vi "FTW-DevUtil-VIDetails.vi"() -> ()   [LabVIEW 2015]
uses:
  linker/FTW-Linker-LinkerInfoStructure.ctl
  linker/FTW-Linker-LabVIEWFiletype.ctl
  linker/FTW-Linker-Flags-viflags2.ctl
  linker/FTW-Linker-Flags-wStyle.ctl
  linker/FTW-Linker-Flags-buttons.ctl
  linker/FTW-Linker-Flags-iState.ctl
  linker/FTW-Linker-Flags-iStyle.ctl
  linker/FTW-Linker-Flags-viflags.ctl
  src/reflection/FTW-Reflection-Types.ctl
panel:
  in  "ScanCLFN":bool=TRUE
  out "CLFN Progress...":dbl(slide) scale=0.0..1.0
  out "Loading Progress...":dbl(slide) scale=0.0..1.0
  in  "Tab":T1(tab)
  in  "Target to Scan":T2(radio)
  out "All Contexts":string[](array[string])
  in  "Context Filter":string="My\\sComputer | XNode | .*"
  out "VIs":T3(array[cluster]) {"SaveVersion" format="%08x"; "FPFlags" format="%08x"; "BDFlags" format="%08x"; "Complexity" format="%.1f"; "HistoryRevision" format="rev %d"; "CompileTime" format="Compile: %dmsec"; "NumCallers" format="%d callers"; "CodeSize" format="BD: %06.1p"; "FPSize" format="FP: %06.1p"}
  in  "Order By":T4(ring)
  out "Controls":T5(array[cluster]) {"HistoryRevision" format="rev %d"; "Callers" format="%d callers"; "FPSize" format="FP %.1p"}
  in  "OrderByDocs":T6(ring) caption="Order By"
  out "VIDocs":T7(array[cluster])
  in  "ContextFilterDocs":string="My\\sComputer | XNode | .*"
  out "All Prototypes":string
  out "CLFNs":T8(array[cluster])
  out "All Links":cluster{"Name":string, "Path":string}[](array[cluster])
  out "LinkerInfo":T9[](array[typedef]) {"iState" format="%08x"; "iStyle" format="%08x"; "wStyle" format="%08x"; "buttons" format="%08x"; "viflags" format="%08x"; "viflags2" format="%08x"}
  out "ExtendedLinkerInfo":T11(array[cluster])
  out "Hover Tip":string
  out "Array":T12(array[cluster]) {"Percentage" format="%.3f%%"}
  in  "Check Coverage":bool
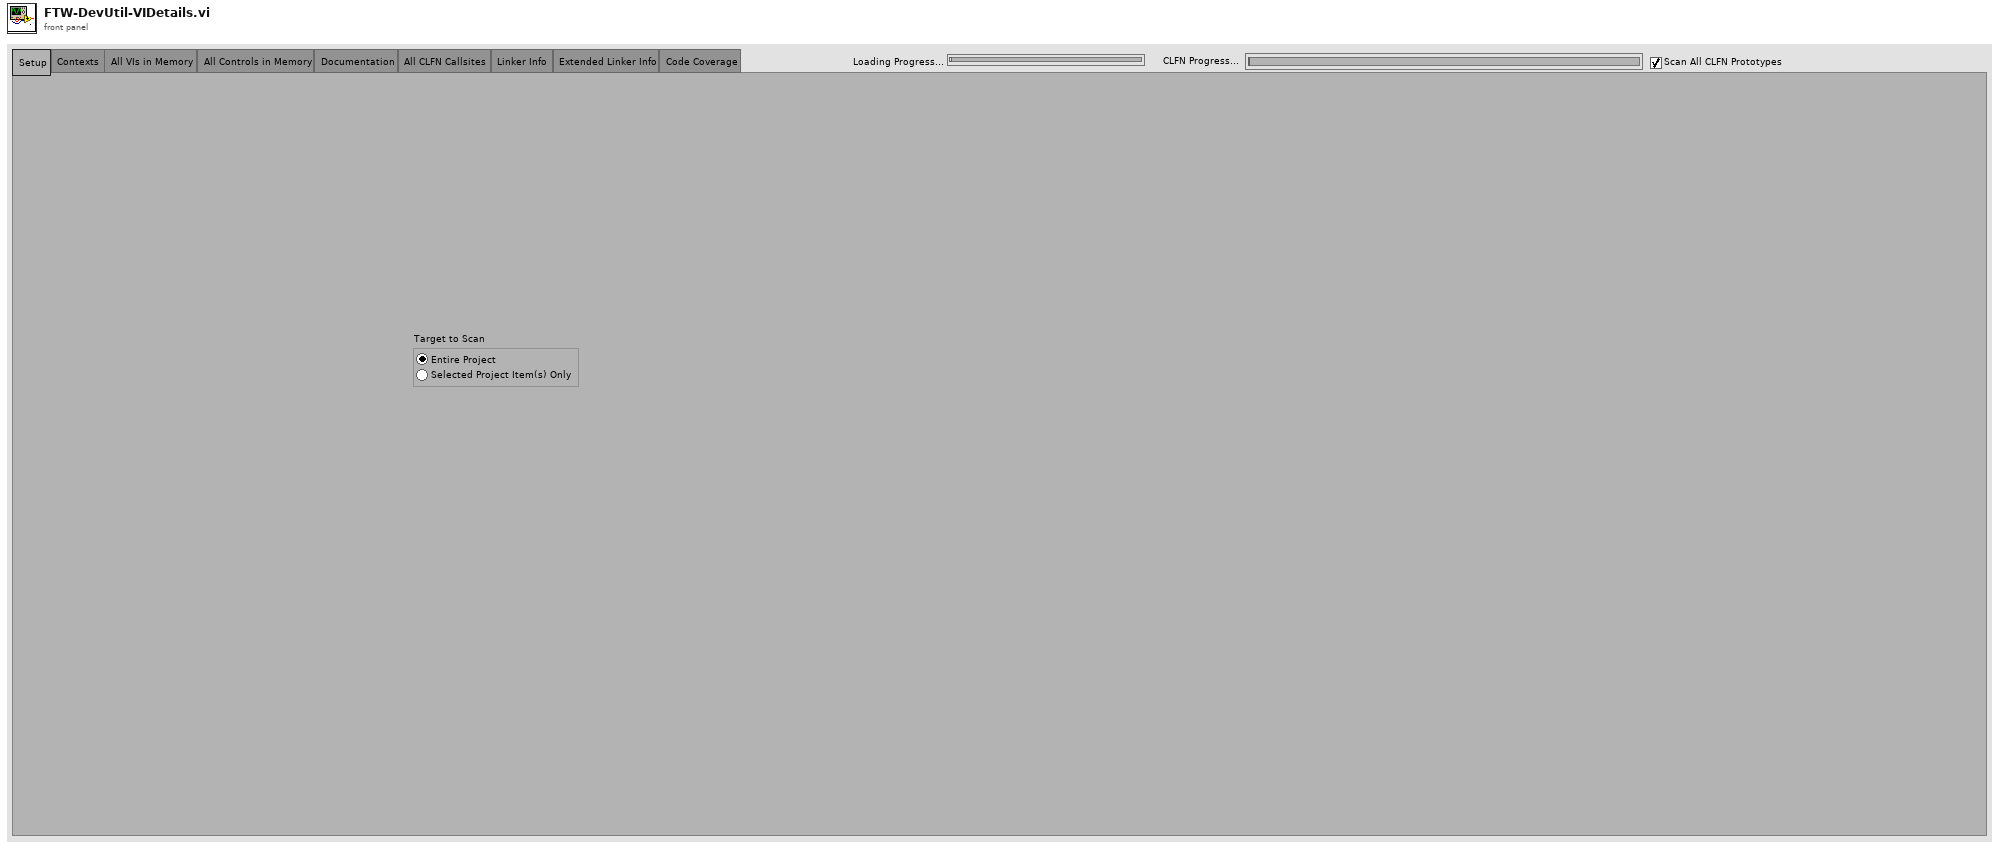
[diagram p1: front panel]
types:
  T1 = enum32{"Setup", "Contexts", "All VIs in Memory", "All Controls in Memory", "Documentation", "All CLFN Callsites", "Linker Info", "Extended Linker Info", "Code Coverage"}
  T2 = enum32{"Entire Project", "Selected Project Item Only"}
  T3 = cluster{"VIRef":refnum<vi>, "Context":string, "Name":string, "FPSize":u32, "CodeSize":u32, "NumCallers":i32, "CompileTime":i32, "Execution":string, "UnexpectedConfig":bool, "ShowRunButton":bool, "ShowRunContButton":bool, "HistoryRevision":u32, "Complexity":sgl, "BDFlags":u32, "FPFlags":u32, "SaveVersion":u32}[]
  T4 = enum16{"Application Context", "Num Callers", "Complexity", "Diagram Size", "FP Size", "Compile Time", "Revisions", "Execution Settings"}
  T5 = cluster{"VIRef":refnum<vi>, "Context":string, "VI":string, "FPSize":u32, "Callers":i32, "SeparateCompiled":bool, "HistoryRevision":u32}[]
  T6 = enum16{"Name", "ConPane Style", "Required Terminals", "Recommended Terminals", "Total Terminals"}
  T7 = cluster{"VIRef":refnum<vi>, "Icon":picture, "Name":string, "HasTags":bool, "VIDescription":string, "Icon16":picture, "IconMono":picture, "OnlineHelp":bool, "ConPane":u32, "Context":string, "InReq":u32, "OutReq":u32, "InRec":u32, "OutRec":u32, "InOpt":u32, "OutOpt":u32, "InDD":u32, "OutDD":u32, "Wired Terms":u32, "WindowTitle":string, "CustomTitle":bool}[]
  T8 = cluster{"CLFNRef":refnum<vi>, "VI":string, "Function":string, "Prototype":string, "CallConv":u32, "LibraryPath":path, "AnyThread":bool, "Dynamic":bool, "ErrCheckLevel":u32, "Reserve":string, "Unreserve":string, "Abort":string, "Prealloc":bool[], "Err":string}[]
  T9 = typedef "FTW-Linker-LinkerInfoStructure.ctl" = cluster{"path":path, "delimited name":string, "Filetype":T10, "iState":u32, "iStyle":u16, "wStyle":u16, "buttons":u16, "viflags":u32, "viflags2":u32, "links":u32[]}
  T10 = typedef "FTW-Linker-LabVIEWFiletype.ctl" = enum32{"Invalid file", "Unknown type", "VI", "Control", "PolyVI", "Project", "Library", "LVClass", "XControl", "XNode", "Shared Library", "dotNET assembly", "ActiveX interface", "CIN", "Run-time menu", "Palette menu", "Help file", "LLB", "XNode Edit Dependency", "LVClass Private Data", "Statechart", "MathScript .m file", "Ladder Diagram", "Packed Project Lib", "XNode Build Dependency"}
  T11 = cluster{"Name":string, "Type":string, "Flags":bool[], "VIRef":refnum<vi>}[]
  T12 = cluster{"Info":bool, "Percentage":dbl, "Path":string}[]
  T13 = typedef "FTW-Linker-Flags-viflags.ctl" = cluster{"Broken Wire":bool, "Broken Node":bool, "Missing SubVI Link":bool, "Broken SubVI":bool, "Not Reservable":bool, "Reentrant":bool, "Close afterward if originally closed":bool, "Reentrant (shared clones)":bool, "Load Front Panel when opened":bool, "Block Diagram not available":bool, "Show front panel when loaded":bool, "Must Call Parent contract broken":bool, "Suspend when called":bool, "Locked":bool, "Run when opened":bool, "Show Front Panel when Called":bool, "Could not compile":bool, "Subroutine priority":bool, "Auto-log at finish":bool, "Compiler bug":bool, "Is Typedef":bool, "Is Strict Typedef":bool, "Bad DDO":bool, "Control Editor has unapplied changes":bool, "Boolean 25":bool, "Owning library broken":bool, "Auto preallocate arrays and strings":bool, "Show Evaluation Watermark":bool, "Show Student Watermark":bool, "Insane VI":bool, "PropTypes warnings (maybe diagram disabled)":bool, "PolyVI broken":bool}
  T14 = typedef "FTW-Linker-Flags-iStyle.ctl" = cluster{"Horizonal Scrollbar Enabled":bool, "Vertical Scrollbar Enabled":bool, "Show menu bar":bool, "Show Toolbar when Running":bool, "Show menu bar":bool, "Window run-time position (Centered)":bool, "Window run-time position (Maximized)":bool, "Allow default run-time shortcut menus":bool, "Highlight Enter Button":bool, "Boolean 10":bool, "Maintain window proportions for different resolutions":bool, "Boolean 12":bool, "Boolean 13":bool, "Boolean 14":bool, "Boolean 15":bool, "Boolean 16":bool}
  T15 = typedef "FTW-Linker-Flags-iState.ctl" = cluster{"Retain Wire Values":bool, "Boolean 2":bool, "Boolean 3":bool, "Boolean 4":bool, "Contains CLFN (???)":bool, "Auto-log at finish":bool, "Boolean 7":bool, "Boolean 8":bool, "Boolean 9":bool, "Allow Debugging":bool, "Boolean 11":bool, "Boolean 12":bool, "Boolean 13":bool, "Boolean 14":bool, "Boolean 15":bool, "Print Logging Enabled":bool, "Boolean 17":bool, "Boolean 18":bool, "Boolean 19":bool, "Boolean 20":bool, "Boolean 21":bool, "Boolean 22":bool, "Boolean 23":bool, "Locked":bool, "Boolean 25":bool, "Boolean 26":bool, "Boolean 27":bool, "Boolean 28":bool, "Boolean 29":bool, "Has Breakpoint":bool, "Allow Debugging":bool, "Boolean 32":bool}
  T16 = typedef "FTW-Linker-Flags-buttons.ctl" = cluster{"Hide Run Button":bool, "Boolean 2":bool, "Boolean 3":bool, "Boolean 4":bool, "Boolean 5":bool, "Hide Run Continuously Button":bool, "Boolean 7":bool, "Hide Abort Button":bool, "Boolean 9":bool, "Boolean 10":bool, "Boolean 11":bool, "Boolean 12":bool, "Is Dynamic Dispatch":bool, "Amalgamation":bool, "Amalgamation Piece":bool, "Dynamic Dispatch Method":bool}
  T17 = typedef "FTW-Linker-Flags-wStyle.ctl" = cluster{"Modal Window":bool, "Floating Window":bool, "Window has title bar":bool, "Allow user to close window":bool, "Allow user to resize window":bool, "Allow user to minimize window":bool, "Window runs transparently":bool, "Boolean 8":bool, "Boolean 9":bool, "Floating Window":bool, "Hide floating window if LV is not active":bool, "Boolean 12":bool, "Boolean 13":bool, "Boolean 14":bool, "Boolean 15":bool, "Boolean 16":bool}
  T18 = typedef "FTW-Linker-Flags-viflags2.ctl" = cluster{"Tagged and not edited":bool, "Hide Instance VI on Drop":bool, "Is System VI":bool, "Is Visible VI (perhaps in hierwin)":bool, "Is XNode VI":bool, "Template Rename in progress":bool, "Transactions Disabled":bool, "Must Call Parent contract satisfied":bool, "Undo/Redo didn't change types":bool, "TypePropper says OK to inline":bool, "Separate Compiled Code":bool, "Inline SubVI if possible":bool, "Transaction is failing":bool, "Runtime SSE optimization enabled":bool, "Student-only VI":bool, "Evaluation-only VI":bool, "Enable PolyVI type adaptation":bool, "Inline":bool, "Need FPDSO recompile":bool, "Deprecated PolyVI":bool, "VI can pass LVClass to CLFN":bool, "Undo/Redo in progress":bool, "Show PolyVI instance icon":bool, "Show PolyVI instance selector":bool, "Clear indicators when called":bool, "Expand when dropped as a SubVI":bool, "No clone if Instance VI":bool, "Is Class Private Data Control":bool, "Is Instance VI":bool, "Enable automatic error handling":bool, "Remote Panel VI":bool, "Suppress Instance VI Halo":bool}
  T19 = cluster{"App.ContextName":string, "Name":string, "Reference":refnum<vi>}
  T20 = cluster{"App.ContextName":string, string, "vi reference":refnum<vi>}
  T21 = cluster{"App.ContextName":string, "Name":string, "Reference":refnum<vi>}[]
  T22 = cluster{"VIRef":refnum<vi>, "Context":string, "VI":string, "FPSize":u32, "Callers":i32, "SeparateCompiled":bool, "HistoryRevision":u32}
  T23 = cluster{"VIRef":refnum<vi>, "Context":string, "Name":string, "FPSize":u32, "CodeSize":u32, "NumCallers":i32, "CompileTime":i32, "Execution":string, "UnexpectedConfig":bool, "ShowRunButton":bool, "ShowRunContButton":bool, "HistoryRevision":u32, "Complexity":sgl, "BDFlags":u32, "FPFlags":u32, "SaveVersion":u32}
  T24 = cluster{"VIRef":refnum<vi>, "Icon":picture, "Name":string, "HasTags":bool, "VIDescription":string, "Icon16":picture, "IconMono":picture, "OnlineHelp":bool, "ConPane":u32, "Context":string, "InReq":u32, "OutReq":u32, "InRec":u32, "OutRec":u32, "InOpt":u32, "OutOpt":u32, "InDD":u32, "OutDD":u32, "Wired Terms":u32, "WindowTitle":string, "CustomTitle":bool}
  T25 = enum32{"invalid VI type", "Standard VI", "Control VI", "Global VI", "Polymorphic VI", "Configuration VI", "SubSystem", "Facade VI", "Method VI", "Statechart Diagram VI"}
  T26 = typedef "imagedata.ctl" = cluster{"image type":i32, "image depth":i32, "image":u8[], "mask":u8[], "colors":u32[], "Rectangle":cluster{"left":i16, "top":i16, "right":i16, "bottom":i16}}
  T27 = enum16{"Invalid Wire Rule", "Required", "Recommended", "Optional", "Dynamic Dispatch"}[]
  T28 = cluster{"[0]":u32, "[1]":u32, "[2]":u32, "[3]":u32, "[4]":u32, "[5]":u32, "[6]":u32, "[7]":u32}
  T29 = cluster{"HistoryRevision":u32, "FPSize":u32, "Callers":i32, "CodeSize":u32, "CompileTime":i32, "Reentrancy":string, "ExecSystem":enum32{"invalid execution system", "user interface", "standard", "instrument i/o", "data acquisition", "other 1", "other 2", "same as caller"}, "Priority":enum32{"invalid priority", "background priority", "normal priority", "above normal priority", "high priority", "time critical priority", "subroutine"}, "UnexpectedConfig":bool, "Debug":bool, "SeparateCompiled":bool, "AutoErrHand":bool, "Purgative":bool, "ShowRunButton":bool, "ShowRunContButton":bool, "Complexity":sgl, "BDFlags":u32, "FPFlags":u32}
  T30 = cluster{"Name":string, "Path":path, "Reference":refnum<vi>}
  T31 = cluster{"Name":string, "Path":path, "Reference":refnum<vi>}[]
  T32 = typedef "FTW-Reflection-Types.ctl" = enum16{"Unknown", "Void", "Array", "Cluster", "LVObject", "Boolean", "I8", "I16", "I32", "I64", "U8", "U16", "U32", "U64", "SGL", "DBL", "EXT", "CSG", "CDB", "CXT", "FXP", "EnumU8", "EnumU16", "EnumU32", "EnumU64", "SGLwithUnit", "DBLwithUnit", "EXTwithUnit", "CSGwithUnit", "CDBwithUnit", "CXTwithUnit", "String", "Path", "Picture", "Tag", "LVVariant", "Timestamp", "WaveformI8", "WaveformI16", "WaveformI32", "WaveformI64", "WaveformU8", "WaveformU16", "WaveformU32", "WaveformU64", "WaveformSGL", "WaveformDBL", "WaveformEXT", "WaveformCSG", "WaveformCDB", "WaveformCXT", "WaveformDigital", "WaveformUnknownType", "DigitalData", "DynamicData", "ExternalData", "FileByteStream", "TDMStream", "dotNET", "ActiveX", "VIServerReference", "VIReference", "ApplicationInstance", "Menu", "ConnectionDataSocket", "ConnectionVISA", "ConnectionBluetooth", "ConnectionIrDA", "ConnectionTCP", "ConnectionUDP", "ConnectionHTTPClient", "ConnectionFTP", "Occurrence", "Notifier", "Queue", "Rendezvous", "Semaphore", "RTFIFO", "EventPublisher", "EventRegistration", "EventCallback", "DataValueReference", "GenericClass", "GenericClassTag", "GenericClassDeepCopy", "GenericClassFlattened", "GenericClassTagFlattened", "GenericReferenceType", "WindowsRegistry", "OverloadedDatalogRef", "ReferenceUnknownType", "ByteArray", "ConPaneInterface", "FTWObject"}
  T33 = cluster{"Element Name":string, "Element Type":T32, "Element Value":variant}[]
  T34 = cluster{"CLFNRef":refnum<vi>, "VI":string, "Function":string, "Prototype":string, "CallConv":u32, "LibraryPath":path, "AnyThread":bool, "Dynamic":bool, "ErrCheckLevel":u32, "Reserve":string, "Unreserve":string, "Abort":string, "Prealloc":bool[], "Err":string}
  T35 = cluster{"Context":string, "Name":string, "VIDetails":cluster{"VIRef":refnum<vi>, "Context":string, "Name":string, "FPSize":u32, "CodeSize":u32, "NumCallers":i32, "CompileTime":i32, "Execution":string, "UnexpectedConfig":bool, "ShowRunButton":bool, "ShowRunContButton":bool, "HistoryRevision":u32, "Complexity":sgl, "BDFlags":u32, "FPFlags":u32, "SaveVersion":u32}}
  T36 = cluster{"Context":string, "Name":string, "VIDetails":cluster{"VIRef":refnum<vi>, "Context":string, "Name":string, "FPSize":u32, "CodeSize":u32, "NumCallers":i32, "CompileTime":i32, "Execution":string, "UnexpectedConfig":bool, "ShowRunButton":bool, "ShowRunContButton":bool, "HistoryRevision":u32, "Complexity":sgl, "BDFlags":u32, "FPFlags":u32, "SaveVersion":u32}}[]
  T37 = cluster{"NumCallers":i32, "Name":string, "VIDetails":cluster{"VIRef":refnum<vi>, "Context":string, "Name":string, "FPSize":u32, "CodeSize":u32, "NumCallers":i32, "CompileTime":i32, "Execution":string, "UnexpectedConfig":bool, "ShowRunButton":bool, "ShowRunContButton":bool, "HistoryRevision":u32, "Complexity":sgl, "BDFlags":u32, "FPFlags":u32, "SaveVersion":u32}}
  T38 = cluster{"NumCallers":i32, "Name":string, "VIDetails":cluster{"VIRef":refnum<vi>, "Context":string, "Name":string, "FPSize":u32, "CodeSize":u32, "NumCallers":i32, "CompileTime":i32, "Execution":string, "UnexpectedConfig":bool, "ShowRunButton":bool, "ShowRunContButton":bool, "HistoryRevision":u32, "Complexity":sgl, "BDFlags":u32, "FPFlags":u32, "SaveVersion":u32}}[]
  T39 = cluster{"Complexity":sgl, "CodeSize":u32, "VIDetails":cluster{"VIRef":refnum<vi>, "Context":string, "Name":string, "FPSize":u32, "CodeSize":u32, "NumCallers":i32, "CompileTime":i32, "Execution":string, "UnexpectedConfig":bool, "ShowRunButton":bool, "ShowRunContButton":bool, "HistoryRevision":u32, "Complexity":sgl, "BDFlags":u32, "FPFlags":u32, "SaveVersion":u32}}
  T40 = cluster{"Complexity":sgl, "CodeSize":u32, "VIDetails":cluster{"VIRef":refnum<vi>, "Context":string, "Name":string, "FPSize":u32, "CodeSize":u32, "NumCallers":i32, "CompileTime":i32, "Execution":string, "UnexpectedConfig":bool, "ShowRunButton":bool, "ShowRunContButton":bool, "HistoryRevision":u32, "Complexity":sgl, "BDFlags":u32, "FPFlags":u32, "SaveVersion":u32}}[]
  T41 = cluster{"CodeSize":u32, "FPSize":u32, "VIDetails":cluster{"VIRef":refnum<vi>, "Context":string, "Name":string, "FPSize":u32, "CodeSize":u32, "NumCallers":i32, "CompileTime":i32, "Execution":string, "UnexpectedConfig":bool, "ShowRunButton":bool, "ShowRunContButton":bool, "HistoryRevision":u32, "Complexity":sgl, "BDFlags":u32, "FPFlags":u32, "SaveVersion":u32}}
  T42 = cluster{"CodeSize":u32, "FPSize":u32, "VIDetails":cluster{"VIRef":refnum<vi>, "Context":string, "Name":string, "FPSize":u32, "CodeSize":u32, "NumCallers":i32, "CompileTime":i32, "Execution":string, "UnexpectedConfig":bool, "ShowRunButton":bool, "ShowRunContButton":bool, "HistoryRevision":u32, "Complexity":sgl, "BDFlags":u32, "FPFlags":u32, "SaveVersion":u32}}[]
  T43 = cluster{"FPSize":u32, "CodeSize":u32, "VIDetails":cluster{"VIRef":refnum<vi>, "Context":string, "Name":string, "FPSize":u32, "CodeSize":u32, "NumCallers":i32, "CompileTime":i32, "Execution":string, "UnexpectedConfig":bool, "ShowRunButton":bool, "ShowRunContButton":bool, "HistoryRevision":u32, "Complexity":sgl, "BDFlags":u32, "FPFlags":u32, "SaveVersion":u32}}
  T44 = cluster{"FPSize":u32, "CodeSize":u32, "VIDetails":cluster{"VIRef":refnum<vi>, "Context":string, "Name":string, "FPSize":u32, "CodeSize":u32, "NumCallers":i32, "CompileTime":i32, "Execution":string, "UnexpectedConfig":bool, "ShowRunButton":bool, "ShowRunContButton":bool, "HistoryRevision":u32, "Complexity":sgl, "BDFlags":u32, "FPFlags":u32, "SaveVersion":u32}}[]
  T45 = cluster{"CompileTime":i32, "Name":string, "VIDetails":cluster{"VIRef":refnum<vi>, "Context":string, "Name":string, "FPSize":u32, "CodeSize":u32, "NumCallers":i32, "CompileTime":i32, "Execution":string, "UnexpectedConfig":bool, "ShowRunButton":bool, "ShowRunContButton":bool, "HistoryRevision":u32, "Complexity":sgl, "BDFlags":u32, "FPFlags":u32, "SaveVersion":u32}}
  T46 = cluster{"CompileTime":i32, "Name":string, "VIDetails":cluster{"VIRef":refnum<vi>, "Context":string, "Name":string, "FPSize":u32, "CodeSize":u32, "NumCallers":i32, "CompileTime":i32, "Execution":string, "UnexpectedConfig":bool, "ShowRunButton":bool, "ShowRunContButton":bool, "HistoryRevision":u32, "Complexity":sgl, "BDFlags":u32, "FPFlags":u32, "SaveVersion":u32}}[]
  T47 = cluster{"HistoryRevision":u32, "Name":string, "VIDetails":cluster{"VIRef":refnum<vi>, "Context":string, "Name":string, "FPSize":u32, "CodeSize":u32, "NumCallers":i32, "CompileTime":i32, "Execution":string, "UnexpectedConfig":bool, "ShowRunButton":bool, "ShowRunContButton":bool, "HistoryRevision":u32, "Complexity":sgl, "BDFlags":u32, "FPFlags":u32, "SaveVersion":u32}}
  T48 = cluster{"HistoryRevision":u32, "Name":string, "VIDetails":cluster{"VIRef":refnum<vi>, "Context":string, "Name":string, "FPSize":u32, "CodeSize":u32, "NumCallers":i32, "CompileTime":i32, "Execution":string, "UnexpectedConfig":bool, "ShowRunButton":bool, "ShowRunContButton":bool, "HistoryRevision":u32, "Complexity":sgl, "BDFlags":u32, "FPFlags":u32, "SaveVersion":u32}}[]
  T49 = cluster{"Execution":string, "Name":string, "VIDetails":cluster{"VIRef":refnum<vi>, "Context":string, "Name":string, "FPSize":u32, "CodeSize":u32, "NumCallers":i32, "CompileTime":i32, "Execution":string, "UnexpectedConfig":bool, "ShowRunButton":bool, "ShowRunContButton":bool, "HistoryRevision":u32, "Complexity":sgl, "BDFlags":u32, "FPFlags":u32, "SaveVersion":u32}}
  T50 = cluster{"Execution":string, "Name":string, "VIDetails":cluster{"VIRef":refnum<vi>, "Context":string, "Name":string, "FPSize":u32, "CodeSize":u32, "NumCallers":i32, "CompileTime":i32, "Execution":string, "UnexpectedConfig":bool, "ShowRunButton":bool, "ShowRunContButton":bool, "HistoryRevision":u32, "Complexity":sgl, "BDFlags":u32, "FPFlags":u32, "SaveVersion":u32}}[]
  T51 = cluster{"Context":string, "Name":string, "VIDocs":cluster{"VIRef":refnum<vi>, "Icon":picture, "Name":string, "HasTags":bool, "VIDescription":string, "Icon16":picture, "IconMono":picture, "OnlineHelp":bool, "ConPane":u32, "Context":string, "InReq":u32, "OutReq":u32, "InRec":u32, "OutRec":u32, "InOpt":u32, "OutOpt":u32, "InDD":u32, "OutDD":u32, "Wired Terms":u32, "WindowTitle":string, "CustomTitle":bool}}
  T52 = cluster{"Context":string, "Name":string, "VIDocs":cluster{"VIRef":refnum<vi>, "Icon":picture, "Name":string, "HasTags":bool, "VIDescription":string, "Icon16":picture, "IconMono":picture, "OnlineHelp":bool, "ConPane":u32, "Context":string, "InReq":u32, "OutReq":u32, "InRec":u32, "OutRec":u32, "InOpt":u32, "OutOpt":u32, "InDD":u32, "OutDD":u32, "Wired Terms":u32, "WindowTitle":string, "CustomTitle":bool}}[]
  T53 = cluster{"ConPane":u32, "Context":string, "Name":string, "VIDocs":cluster{"VIRef":refnum<vi>, "Icon":picture, "Name":string, "HasTags":bool, "VIDescription":string, "Icon16":picture, "IconMono":picture, "OnlineHelp":bool, "ConPane":u32, "Context":string, "InReq":u32, "OutReq":u32, "InRec":u32, "OutRec":u32, "InOpt":u32, "OutOpt":u32, "InDD":u32, "OutDD":u32, "Wired Terms":u32, "WindowTitle":string, "CustomTitle":bool}}
  T54 = cluster{"ConPane":u32, "Context":string, "Name":string, "VIDocs":cluster{"VIRef":refnum<vi>, "Icon":picture, "Name":string, "HasTags":bool, "VIDescription":string, "Icon16":picture, "IconMono":picture, "OnlineHelp":bool, "ConPane":u32, "Context":string, "InReq":u32, "OutReq":u32, "InRec":u32, "OutRec":u32, "InOpt":u32, "OutOpt":u32, "InDD":u32, "OutDD":u32, "Wired Terms":u32, "WindowTitle":string, "CustomTitle":bool}}[]
  T55 = cluster{u32, u32, "Name":string, "VIDocs":cluster{"VIRef":refnum<vi>, "Icon":picture, "Name":string, "HasTags":bool, "VIDescription":string, "Icon16":picture, "IconMono":picture, "OnlineHelp":bool, "ConPane":u32, "Context":string, "InReq":u32, "OutReq":u32, "InRec":u32, "OutRec":u32, "InOpt":u32, "OutOpt":u32, "InDD":u32, "OutDD":u32, "Wired Terms":u32, "WindowTitle":string, "CustomTitle":bool}}
  T56 = cluster{u32, u32, "Name":string, "VIDocs":cluster{"VIRef":refnum<vi>, "Icon":picture, "Name":string, "HasTags":bool, "VIDescription":string, "Icon16":picture, "IconMono":picture, "OnlineHelp":bool, "ConPane":u32, "Context":string, "InReq":u32, "OutReq":u32, "InRec":u32, "OutRec":u32, "InOpt":u32, "OutOpt":u32, "InDD":u32, "OutDD":u32, "Wired Terms":u32, "WindowTitle":string, "CustomTitle":bool}}[]
  T57 = cluster{"Wired Terms":u32, "Name":string, "VIDocs":cluster{"VIRef":refnum<vi>, "Icon":picture, "Name":string, "HasTags":bool, "VIDescription":string, "Icon16":picture, "IconMono":picture, "OnlineHelp":bool, "ConPane":u32, "Context":string, "InReq":u32, "OutReq":u32, "InRec":u32, "OutRec":u32, "InOpt":u32, "OutOpt":u32, "InDD":u32, "OutDD":u32, "Wired Terms":u32, "WindowTitle":string, "CustomTitle":bool}}
  T58 = cluster{"Wired Terms":u32, "Name":string, "VIDocs":cluster{"VIRef":refnum<vi>, "Icon":picture, "Name":string, "HasTags":bool, "VIDescription":string, "Icon16":picture, "IconMono":picture, "OnlineHelp":bool, "ConPane":u32, "Context":string, "InReq":u32, "OutReq":u32, "InRec":u32, "OutRec":u32, "InOpt":u32, "OutOpt":u32, "InDD":u32, "OutDD":u32, "Wired Terms":u32, "WindowTitle":string, "CustomTitle":bool}}[]
  T59 = cluster{"infoFound":bool, "covPercent":dbl, string}
  T60 = cluster{"infoFound":bool, "covPercent":dbl, string}[]
  T61 = cluster{string, "delimited name":string, "All Flags":bool[], "vi reference":refnum<vi>}
  T62 = cluster{"LibraryPath":path, "VI":string, "Function":string, "CLFN Array Element":cluster{"CLFNRef":refnum<vi>, "VI":string, "Function":string, "Prototype":string, "CallConv":u32, "LibraryPath":path, "AnyThread":bool, "Dynamic":bool, "ErrCheckLevel":u32, "Reserve":string, "Unreserve":string, "Abort":string, "Prealloc":bool[], "Err":string}}
  T63 = cluster{string, "delimited name":string, "All Flags":bool[], "vi reference":refnum<vi>}[]
  T64 = cluster{"LibraryPath":path, "VI":string, "Function":string, "CLFN Array Element":cluster{"CLFNRef":refnum<vi>, "VI":string, "Function":string, "Prototype":string, "CallConv":u32, "LibraryPath":path, "AnyThread":bool, "Dynamic":bool, "ErrCheckLevel":u32, "Reserve":string, "Unreserve":string, "Abort":string, "Prealloc":bool[], "Err":string}}[]
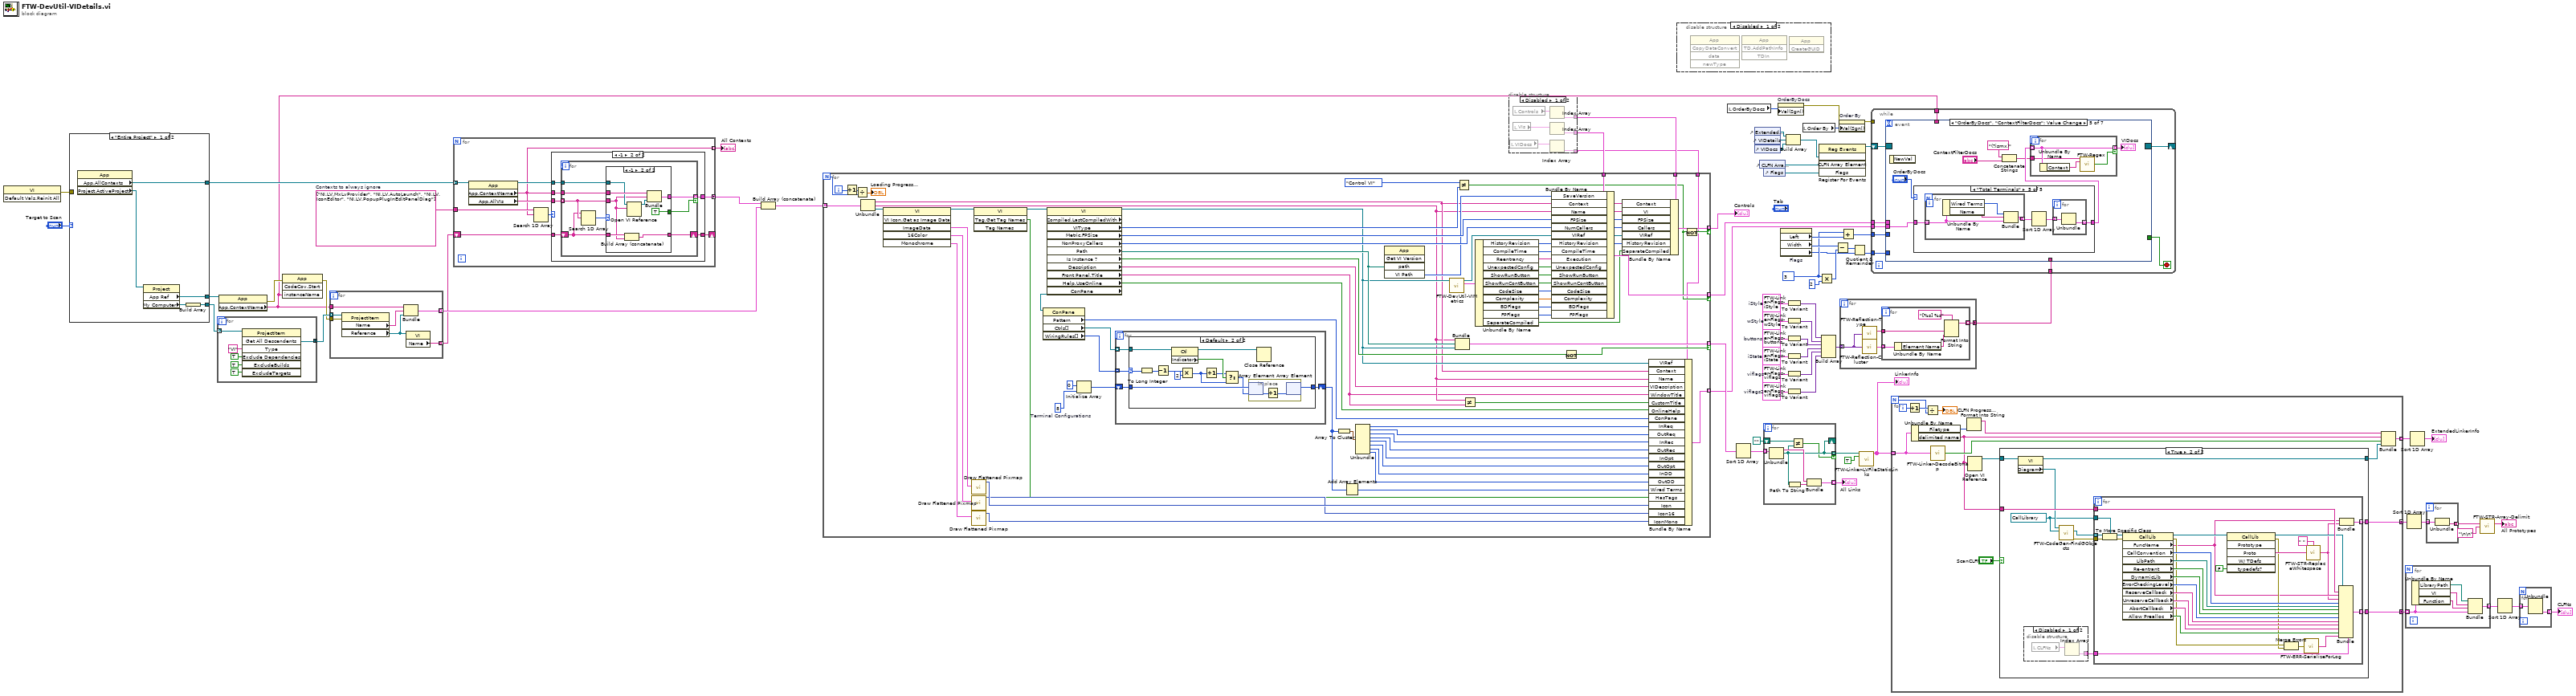
[diagram p0: block diagram]
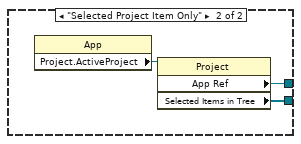
[diagram p3: hidden frame]
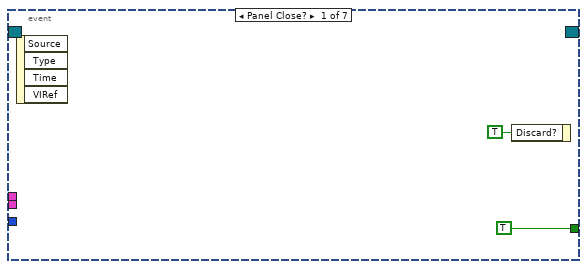
[diagram p8: hidden frame]
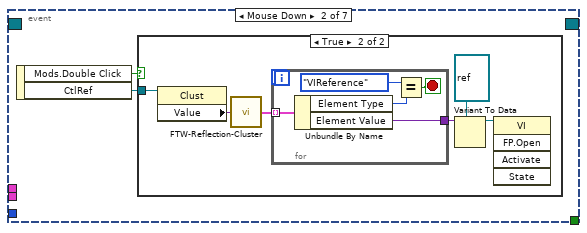
[diagram p9: hidden frame]
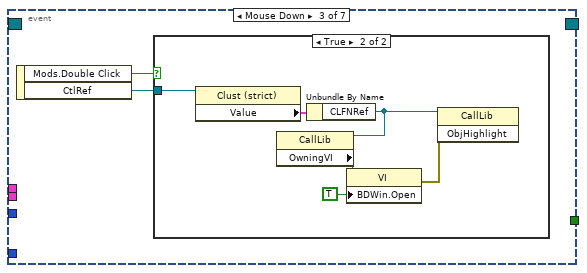
[diagram p11: hidden frame]
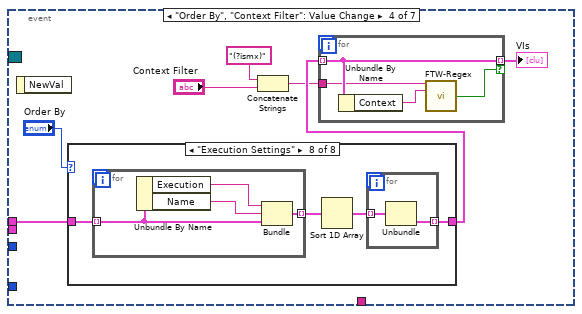
[diagram p13: hidden frame]
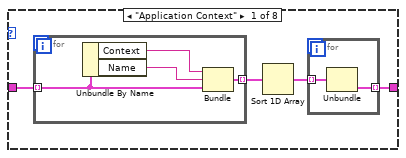
[diagram p14: hidden frame]
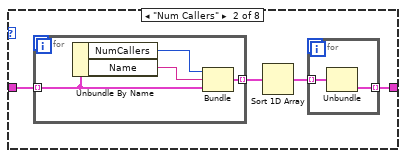
[diagram p15: hidden frame]
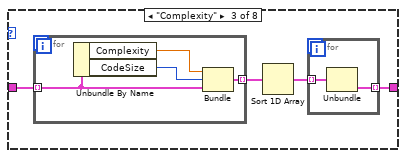
[diagram p16: hidden frame]
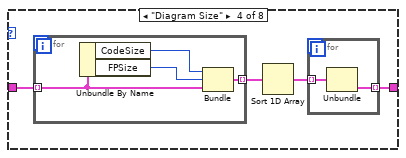
[diagram p17: hidden frame]
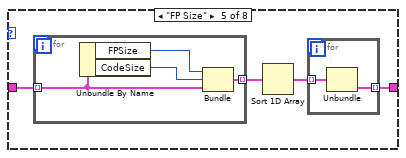
[diagram p18: hidden frame]
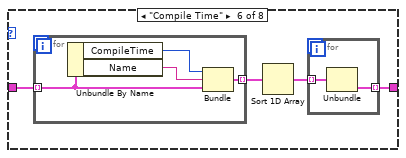
[diagram p19: hidden frame]
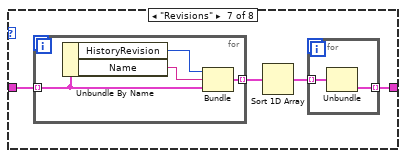
[diagram p20: hidden frame]
diagram:
  w21 = T13 {"Broken Wire"=FALSE, "Broken Node"=FALSE, "Missing SubVI Link"=FALSE, "Broken SubVI"=FALSE, "Not Reservable"=FALSE, "Reentrant"=FALSE, "Close afterward if originally closed"=FALSE, "Reentrant (shared clones)"=FALSE, "Load Front Panel when opened"=FALSE, "Block Diagram not available"=FALSE, "Show front panel when loaded"=FALSE, "Must Call Parent contract broken"=FALSE, "Suspend when called"=FALSE, "Locked"=FALSE, "Run when opened"=FALSE, "Show Front Panel when Called"=FALSE, "Could not compile"=FALSE, "Subroutine priority"=FALSE, "Auto-log at finish"=FALSE, "Compiler bug"=FALSE, "Is Typedef"=FALSE, "Is Strict Typedef"=FALSE, "Bad DDO"=FALSE, "Control Editor has unapplied changes"=FALSE, "Boolean 25"=FALSE, "Owning library broken"=FALSE, "Auto preallocate arrays and strings"=FALSE, "Show Evaluation Watermark"=FALSE, "Show Student Watermark"=FALSE, "Insane VI"=FALSE, "PropTypes warnings (maybe diagram disabled)"=FALSE, "PolyVI broken"=FALSE}  # viflags
  w25 = T14 {"Horizonal Scrollbar Enabled"=FALSE, "Vertical Scrollbar Enabled"=FALSE, "Show menu bar"=FALSE, "Show Toolbar when Running"=FALSE, "Show menu bar"=FALSE, "Window run-time position (Centered)"=FALSE, "Window run-time position (Maximized)"=FALSE, "Allow default run-time shortcut menus"=FALSE, "Highlight Enter Button"=FALSE, "Boolean 10"=FALSE, "Maintain window proportions for different resolutions"=FALSE, "Boolean 12"=FALSE, "Boolean 13"=FALSE, "Boolean 14"=FALSE, "Boolean 15"=FALSE, "Boolean 16"=FALSE}  # iStyle
  w22 = T15 {"Retain Wire Values"=FALSE, "Boolean 2"=FALSE, "Boolean 3"=FALSE, "Boolean 4"=FALSE, "Contains CLFN (???)"=FALSE, "Auto-log at finish"=FALSE, "Boolean 7"=FALSE, "Boolean 8"=FALSE, "Boolean 9"=FALSE, "Allow Debugging"=FALSE, "Boolean 11"=FALSE, "Boolean 12"=FALSE, "Boolean 13"=FALSE, "Boolean 14"=FALSE, "Boolean 15"=FALSE, "Print Logging Enabled"=FALSE, "Boolean 17"=FALSE, "Boolean 18"=FALSE, "Boolean 19"=FALSE, "Boolean 20"=FALSE, "Boolean 21"=FALSE, "Boolean 22"=FALSE, "Boolean 23"=FALSE, "Locked"=FALSE, "Boolean 25"=FALSE, "Boolean 26"=FALSE, "Boolean 27"=FALSE, "Boolean 28"=FALSE, "Boolean 29"=FALSE, "Has Breakpoint"=FALSE, "Allow Debugging"=FALSE, "Boolean 32"=FALSE}  # iState
  w23 = T16 {"Hide Run Button"=FALSE, "Boolean 2"=FALSE, "Boolean 3"=FALSE, "Boolean 4"=FALSE, "Boolean 5"=FALSE, "Hide Run Continuously Button"=FALSE, "Boolean 7"=FALSE, "Hide Abort Button"=FALSE, "Boolean 9"=FALSE, "Boolean 10"=FALSE, "Boolean 11"=FALSE, "Boolean 12"=FALSE, "Is Dynamic Dispatch"=FALSE, "Amalgamation"=FALSE, "Amalgamation Piece"=FALSE, "Dynamic Dispatch Method"=FALSE}  # buttons
  w24 = T17 {"Modal Window"=FALSE, "Floating Window"=FALSE, "Window has title bar"=FALSE, "Allow user to close window"=FALSE, "Allow user to resize window"=FALSE, "Allow user to minimize window"=FALSE, "Window runs transparently"=FALSE, "Boolean 8"=FALSE, "Boolean 9"=FALSE, "Floating Window"=FALSE, "Hide floating window if LV is not active"=FALSE, "Boolean 12"=FALSE, "Boolean 13"=FALSE, "Boolean 14"=FALSE, "Boolean 15"=FALSE, "Boolean 16"=FALSE}  # wStyle
  w20 = T18 {"Tagged and not edited"=FALSE, "Hide Instance VI on Drop"=FALSE, "Is System VI"=FALSE, "Is Visible VI (perhaps in hierwin)"=FALSE, "Is XNode VI"=FALSE, "Template Rename in progress"=FALSE, "Transactions Disabled"=FALSE, "Must Call Parent contract satisfied"=FALSE, "Undo/Redo didn't change types"=FALSE, "TypePropper says OK to inline"=FALSE, "Separate Compiled Code"=FALSE, "Inline SubVI if possible"=FALSE, "Transaction is failing"=FALSE, "Runtime SSE optimization enabled"=FALSE, "Student-only VI"=FALSE, "Evaluation-only VI"=FALSE, "Enable PolyVI type adaptation"=FALSE, "Inline"=FALSE, "Need FPDSO recompile"=FALSE, "Deprecated PolyVI"=FALSE, "VI can pass LVClass to CLFN"=FALSE, "Undo/Redo in progress"=FALSE, "Show PolyVI instance icon"=FALSE, "Show PolyVI instance selector"=FALSE, "Clear indicators when called"=FALSE, "Expand when dropped as a SubVI"=FALSE, "No clone if Instance VI"=FALSE, "Is Class Private Data Control"=FALSE, "Is Instance VI"=FALSE, "Enable automatic error handling"=FALSE, "Remote Panel VI"=FALSE, "Suppress Instance VI Halo"=FALSE}  # viflags2
  w42 = 3 ("x")
  w67 = string[] ["NI.LV.MxLvProvider", "NI.LV.AutoLaunch", "NI.LV.IconEditor", "NI.LV.PopupPlugInEditPanelDiag"]  # Contexts to always ignore
  n1 = invoke class="VI" method="Default Vals.Reinit All"() -> (error out=w18:errorcluster)  [unwired: 3 in, 2 out]
  n2 = case shown="\"Entire Project\"" "Target to Scan" {
    tunnel: [w78 _] -> w69
    tunnel: [w74 w80] -> w59
    tunnel: [w75 w79] -> w57
    tunnel: w18 -> [_ _]
    frame "Entire Project" {
      n3 = property class="App"() -> ("App.AllContexts"=w78:refnum<vi>[], "Project.ActiveProject"=w77:refnum<vi>)  [unwired: 2 in, 2 out]
      n4 = property class="Project"(reference=w77) -> ("App Ref"=w75:refnum<vi>, "My Computer"=w76:refnum<vi>)  [unwired: 1 in, 2 out]
      n5 = Build Array(w76) -> (w74:refnum<vi>[])
    }
    frame "Selected Project Item Only" {
      n6 = property class="App"() -> ("Project.ActiveProject"=w81:refnum<vi>)  [unwired: 2 in, 2 out]
      n7 = property class="Project"(reference=w81) -> ("App Ref"=w79:refnum<vi>, "Selected Items in Tree"=w80:refnum<vi>[])  [unwired: 1 in, 2 out]
    }
  }
  n8 = for {
    tunnel: w59 -> [w87] mode=indexing
    tunnel: [w86] -> w58 mode=concatenating
    n9 = invoke class="ProjectItem" method="Get All Descendents"(reference=w87, "Type"="VI", "Exclude Dependencies"=TRUE ("ExcludeDependencies"), "ExcludeBuilds"=TRUE, "ExcludeTargets"=TRUE) -> ("All Descendents"=w86:refnum<vi>[])  [unwired: 2 in, 6 out]
  }
  n10 = property class="App"(reference=w57) -> (error out=w8:errorcluster, "App.ContextName"=w6:string)  [unwired: 1 in, 1 out]
  n11 = invoke class="App" method="CodeCov.Start"(error in=w8, "instanceName"=w6) -> (error out=w7:errorcluster)  [unwired: 2 in, 3 out]
  n12 = for {
    tunnel: w58 -> [w94] mode=indexing
    tunnel: w6 -> [w93]
    tunnel: [w92] -> w56 mode=indexing
    tunnel: [w89] -> w47 mode=indexing
    tunnel: w7 -> [w88]
    n13 = property class="ProjectItem"(reference=w94, error in=w88) -> ("Name"=w91:string, "Reference"=w90:refnum<vi>)  [unwired: 2 out]
    n14 = Bundle("App.ContextName"=w93, "Name"=w91, "Reference"=w90) -> (w92:T19)  [unwired: 1 in]
    n15 = property class="VI"(reference=w90) -> ("Name"=w89:string)  [unwired: 1 in, 2 out]
  }
  n16 = for {
    tunnel: w69 -> [w102] mode=indexing
    tunnel: [w95] -> w68 mode=indexing
    tunnel: [w99] -> w54 mode=concatenating
    tunnel: w67 -> [w101]
    shift-right: [w96] -> _
    shift-left: w47 -> [w97]
    n17 = property class="App"(reference=w102) -> (reference out=w100:refnum<vi>, "App.ContextName"=w95:string, "App.AllVIs"=w103:string[])  [unwired: 1 in, 1 out]
    n18 = Search 1D Array(1D array=w101, element=w95) -> (index of element=w98:i32)  [unwired: 1 in]
    n19 = case shown="-1" w98 {
      tunnel: w103 -> [_ w110]
      tunnel: w95 -> [_ w109]
      tunnel: w100 -> [_ w108]
      tunnel: [_ w107] -> w99
      tunnel: w97 -> [w104 w105]
      tunnel: [w104 w106] -> w96
      frame Default {
      }
      frame -1 {
        n20 = for {
          tunnel: w109 -> [w118]
          tunnel: w110 -> [w115] mode=indexing
          tunnel: [w117] -> w107 mode=indexing if=w111
          tunnel: w108 -> [w116]
          shift-right: [w113] -> w106
          shift-left: w105 -> [w112]
          n21 = Search 1D Array(1D array=w112, element=w115) -> (index of element=w114:i32)  [unwired: 1 in]
          n22 = case shown="-1" w114 {
            tunnel: w118 -> [_ w127]
            tunnel: [_ w126] -> w117
            tunnel: w116 -> [_ w124]
            tunnel: w115 -> [_ w121]
            tunnel: [w119 w122] -> w113
            tunnel: w112 -> [w119 w123]
            tunnel: [_ TRUE] -> w111
            frame 0, Default {
            }
            frame -1 {
              n23 = Build Array (concatenate)(w123, w121) -> (w122:string[])
              n24 = Open VI Reference(application reference (local)=w124, vi path=w121) -> (vi reference=w125:refnum<vi>)  [unwired: 4 in, 1 out]
              n25 = Bundle("App.ContextName"=w127, w121, "vi reference"=w125) -> (w126:T20)  [unwired: 1 in]
            }
          }
        }
      }
    }
  }
  "All Contexts" <- w68
  n26 = Build Array (concatenate)(w54, w56) -> (w55:T21)
  n27 = disable-structure shown="Disabled" {
    disable-tunnel: [w132 _] -> w73
    disable-tunnel: [w130 _] -> w61
    disable-tunnel: [w128 _] -> w5
    frame Disabled {
      n28 = local read "VIDocs"() -> (w129:T7)
      n29 = local read "Controls"() -> (w131:T5)
      n30 = local read "VIs"() -> (w133:T3)
      n31 = Index Array(array=w131) -> (element=w130:T22)  [unwired: 1 in]
      n32 = Index Array(array=w133) -> (element=w132:T23)  [unwired: 1 in]
      n33 = Index Array(array=w129) -> (element=w128:T24)  [unwired: 1 in]
    }
    frame Enabled {
    }
  }
  n34 = for {
    N -> [w195]
    tunnel: [w203] -> w65 mode=indexing if=w173
    tunnel: w73 -> [w202]
    tunnel: w55 -> [w201] mode=indexing
    tunnel: w61 -> [w198]
    tunnel: [w197] -> w60 mode=indexing if=w196
    tunnel: [w189] -> w53 mode=indexing if=w171
    tunnel: w5 -> [w169]
    tunnel: [w166] -> w1 mode=indexing
    i -> [w194]
    w150 = 8  # Terminal Configurations
    n35 = Increment(x=w194) -> (x+1=w192:i32)
    n36 = Divide(x=w192, y=w195) -> (x/y=→"Loading Progress...":dbl)
    n37 = Unbundle(w201) -> ("App.ContextName"=w153:string, "Name"=w136:string, "Reference"=w170:refnum<vi>)
    n38 = invoke class="VI" method="VI Icon.Get as Image Data"(reference=w170) -> (reference out=w159:refnum<vi>, "ImageData"=w165:T26, "16Color"=w163:T26, "Monochrome"=w160:T26)  [unwired: 5 in, 2 out]
    n39 = call <vilib>:"Draw Flattened Pixmap.vi"("image data"=w165) -> ("new picture"=w164:picture)  [unwired: 8 in]
    n40 = call <vilib>:"Draw Flattened Pixmap.vi"("image data"=w163) -> ("new picture"=w162:picture)  [unwired: 8 in]
    n41 = call <vilib>:"Draw Flattened Pixmap.vi"("image data"=w160) -> ("new picture"=w161:picture)  [unwired: 8 in]
    n42 = invoke class="VI" method="Tag.Get Tag Names"(reference=w159) -> (reference out=w158:refnum<vi>, "Tag.Get Tag Names"=w157:bool)  [unwired: 3 in, 2 out]
    n43 = property class="VI" props=["Compiled.LastCompiledWith", "VIType", "Metric.FPSize", "NonProxyCallers", "Path", "Is Instance ?", "Description", "Front Panel.Title", "Help.UseOnline", "ConPane"](reference=w158) -> (reference out=w168:refnum<vi>, "VIType"=w200:T25, "Metric.FPSize"=w191:u32, "NonProxyCallers"=w190:i32, "Path"=w175:path, "Is Instance ?"=w172:bool, "Description"=w167:string, "Front Panel.Title"=w135:string, "Help.UseOnline"=w156:bool, "ConPane"=w155:refnum<vi>)  [unwired: 1 in, 2 out]
    n44 = property class="ConPane"(reference=w155) -> ("Pattern"=w154:u32, "Ctrls[]"=w152:refnum<vi>[], "WiringRules[]"=w151:T27)  [unwired: 1 in, 2 out]
    n45 = Initialize Array(u32 0 ("element"), w150) -> (w148:u32[])
    n46 = for {
      tunnel: w152 -> [w207] mode=indexing
      tunnel: w151 -> [w206] mode=indexing
      shift-right: [w204] -> w138
      shift-left: w148 -> [w205]
      n47 = case shown="Default" w206 {
        selector: w206 -> [_ w220]
        tunnel: w207 -> [_ w214]
        tunnel: w205 -> [w208 w215]
        tunnel: [w208 w216] -> w204
        frame "Invalid Wire Rule" {
        }
        frame Default {
          n48 = To Long Integer(number=w220) -> (32bit integer=w219:i32)
          n49 = Decrement(x=w219) -> (x-1=w218:i32)
          n50 = property class="Ctl"(reference=w214) -> (reference out=w213:refnum<vi>, "Indicator"=w212:bool)  [unwired: 1 in, 1 out]
          n51 = Multiply(x=w218, y=2) -> (x*y=w211:i32)
          n52 = Increment(x=w211) -> (x+1=w210:i32)
          n53 = Select(t=w210, s=w212, f=w211) -> (s? t:f=w209:i32)
          n54 = in-place {
            n55 = in-place-array #1(w215, w209) -> (w222:u32)
            n56 = Increment(x=w222) -> (x+1=w221:u32)
            n57 = in-place-array #1(w221) -> (w216:u32[])  [unwired: 1 out]
          }
          n58 = Close Reference(reference=w213) -> ()  [unwired: 1 in, 1 out]
        }
      }
    }
    n59 = Array To Cluster(array=w138) -> (cluster=w147:T28)
    n60 = Add Array Elements(numeric array=w138) -> (sum=w137:u32)
    n61 = Unbundle(w147) -> ("[0]"=w146:u32, "[1]"=w145:u32, "[2]"=w144:u32, "[3]"=w143:u32, "[4]"=w142:u32, "[5]"=w141:u32, "[6]"=w140:u32, "[7]"=w139:u32)
    n62 = invoke class="App" method="Get VI Version"("path"=w175) -> ("VI Path"=w174:u32)  [unwired: 4 in, 4 out]
    n63 = call "FTW-DevUtil-VIMetrics.vi"("VI Ref"=w168) -> ("VI Ref out"=w176:refnum<vi>, "VI Metrics"=w188:T29)  [unwired: 12 in, 1 out]
    n64 = Bundle("Name"=w136, "Path"=w175, "Reference"=w168) -> (w189:T30)  [unwired: 1 in]
    n65 = Not Equal?(x=T25."Control VI", y=w200) -> (x != y?=w173:bool)
    n66 = Not Equal?(x=w136, y=w135) -> (x != y?=w134:bool)
    n67 = Unbundle By Name(w188) -> ("HistoryRevision"=w177:u32, "CompileTime"=w187:i32, "Reentrancy"=w186:string, "UnexpectedConfig"=w185:bool, "ShowRunButton"=w184:bool, "ShowRunContButton"=w183:bool, "CodeSize"=w179:u32, "Complexity"=w182:sgl, "BDFlags"=w181:u32, "FPFlags"=w180:u32, "SeparateCompiled"=w178:bool)
    n68 = Bundle By Name(cluster=w202, "SaveVersion"=w174, "Context"=w153, "Name"=w136, "FPSize"=w191, "NumCallers"=w190, "VIRef"=w176, "HistoryRevision"=w177, "CompileTime"=w187, "Execution"=w186, "UnexpectedConfig"=w185, "ShowRunButton"=w184, "ShowRunContButton"=w183, "CodeSize"=w179, "Complexity"=w182, "BDFlags"=w181, "FPFlags"=w180) -> (w203:T23)
    n69 = Not(x=w172) -> (.not. x?=w171:bool)
    n70 = Bundle By Name(cluster=w198, "Context"=w153, "VI"=w136, "FPSize"=w191, "Callers"=w190, "VIRef"=w176, "HistoryRevision"=w177, "SeparateCompiled"=w178) -> (w197:T22)
    n71 = Bundle By Name(cluster=w169, "VIRef"=w168, "Context"=w153, "Name"=w136, "VIDescription"=w167, "WindowTitle"=w135, "CustomTitle"=w134, "OnlineHelp"=w156, "ConPane"=w154, "InReq"=w146, "OutReq"=w145, "InRec"=w144, "OutRec"=w143, "InOpt"=w142, "OutOpt"=w141, "InDD"=w140, "OutDD"=w139, "Wired Terms"=w137, "HasTags"=w157, "Icon"=w164, "Icon16"=w162, "IconMono"=w161) -> (w166:T24)
    n72 = Not(x=w173) -> (.not. x?=w196:bool)
  }
  "Controls" <- w60
  n73 = disable-structure shown="Disabled" {
    frame Disabled {
      n74 = invoke class="App" method="CopyDataConvert"() -> ()  [unwired: 5 in, 5 out]
      n75 = invoke class="App" method="TD.AddPathInfo"() -> ()  [unwired: 4 in, 4 out]
      n76 = invoke class="App" method="CreateGUID"() -> ()  [unwired: 3 in, 3 out]
    }
    frame Enabled {
    }
  }
  n77 = local read "OrderByDocs"() -> (w3:T6)
  n78 = Sort 1D Array(array=w53) -> (sorted array=w51:T31)
  n79 = control-ref of="Extended Linker Info"() -> (w28:refnum<vi>)
  n80 = control-ref of="VIDetails"() -> (w27:refnum<vi>)
  n81 = control-ref of="VIDocs"() -> (w4:refnum<vi>)
  n82 = control-ref of="CLFN Array Element"() -> (w62:refnum<vi>)
  n83 = control-ref of="Flags"() -> (w46:refnum<vi>)
  n84 = for {
    tunnel: w51 -> [w229] mode=indexing
    tunnel: [w224] -> w50 mode=indexing if=w223
    tunnel: [w226] -> w49 mode=indexing
    shift-right: [w224] -> _
    shift-left: path "" -> [w225]
    n85 = Unbundle(w229) -> ("Name"=w228:string, "Path"=w224:path)  [unwired: 1 out]
    n86 = Path To String(path=w224) -> (string=w227:string)
    n87 = Not Equal?(x=w225, y=w224) -> (x != y?=w223:bool)
    n88 = Bundle("Name"=w228, w227) -> (w226:cluster{"Name":string, string})  [unwired: 1 in]
  }
  "All Links" <- w49
  n89 = property on="OrderByDocs" class="Enum (strict)"("Val(Sgnl)"=w3) -> (error out=w2:errorcluster)  [unwired: 2 in, 1 out]
  n90 = property on="Flags" class="Arr (strict)"() -> ("Left"=w45:i32, "Width"=w43:u32, "Number of Columns"=w38:u32)  [unwired: 2 in, 2 out]
  n91 = Build Array(w28, w27, w4) -> (w26:refnum<vi>[])
  n92 = To Variant(anything=w25) -> (Variant=w36:variant)
  n93 = To Variant(anything=w24) -> (Variant=w35:variant)
  n94 = To Variant(anything=w23) -> (Variant=w34:variant)
  n95 = To Variant(anything=w22) -> (Variant=w33:variant)
  n96 = To Variant(anything=w21) -> (Variant=w32:variant)
  n97 = To Variant(anything=w20) -> (Variant=w31:variant)
  n98 = local read "Order By"() -> (w63:T4)
  n99 = register-events(w26, w62, w46) -> (reference out=w66:refnum<event-registration>)  [unwired: 2 in, 1 out]
  n100 = Multiply(x=w42, y=2) -> (x*y=w40:i32)
  n101 = Build Array(w36, w35, w34, w33, w32, w31) -> (w30:variant[])
  n102 = Subtract(x=w43, y=w40) -> (x-y=w39:u32)
  n103 = property on="Order By" class="Enum (strict)"(error in=w2, "Val(Sgnl)"=w63) -> (error out=w64:errorcluster)  [unwired: 1 in, 1 out]
  n104 = for {
    tunnel: w30 -> [w231] mode=indexing
    tunnel: [w232] -> w29 mode=concatenating
    n105 = call "FTW-Reflection-Type.vi"("Anything"=w231) -> ("Data Name"=w230:string)  [unwired: 12 in, 2 out]
    n106 = call "FTW-Reflection-Cluster.vi"("Cluster"=w231) -> ("Cluster Elements"=w233:T33)  [unwired: 14 in]
    n107 = for {
      tunnel: w233 -> [w238] mode=indexing
      tunnel: [w234] -> w232 mode=indexing
      tunnel: w230 -> [w237]
      n108 = Unbundle By Name(w238) -> ("Element Name"=w235:string)
      n109 = Format Into String(format string="[%s] %s", w237, w235) -> (resulting string=w234:string)  [unwired: 2 in, 1 out]
    }
  }
  n110 = Add(x=w42, y=w45) -> (x+y=w44:i32)
  n111 = Quotient & Remainder(x=w39, y=w38) -> (floor(x/y)=w37:u32)  [unwired: 1 out]
  n112 = call "FTW-Linker-LVFileStaticLinks.vi"("LabVIEW Files"=w50, "Recursive"=TRUE) -> ("LinkerInfo"=w17:T9[])  [unwired: 12 in, 1 out]
  "LinkerInfo" <- w17
  n113 = while {
    shift-right: [w245] -> _
    shift-left: w66 -> [w246]
    tunnel: w65 -> [w244]
    tunnel: w64 -> [_]
    tunnel: w44 -> [w243]
    tunnel: w37 -> [w242]
    tunnel: w29 -> [w241]
    tunnel: w6 -> [w240]
    tunnel: w1 -> [w239]
    stop <- w247 stop-if-true
    n114 = event shown="[4] \"OrderByDocs\", \"ContextFilterDocs\": Value Change" {
      selector: w246 -> [_ _ _ _ _ _ _]
      dyn-events: [_ _ _ _ _ _ _] -> w245
      timeout: _ -> [_ _ _ _ _ _ _]
      tunnel: [TRUE _ _ _ _ _ _] -> w247
      tunnel: w244 -> [_ _ _ w277 _ _ _]
      tunnel: w243 -> [_ _ _ _ _ _ _]
      tunnel: w242 -> [_ _ _ _ _ _ _]
      tunnel: w241 -> [_ _ _ _ _ _ w450]
      tunnel: w240 -> [_ _ _ _ _ w436 _]
      tunnel: w239 -> [_ _ _ _ w364 _ _]
      event Panel Close? {
        n115 = event-data() -> ()  [unwired: 1 in, 4 out]
        n116 = event-data("Discard?"=TRUE) -> ()  [unwired: 1 in, 1 out]
      }
      event Mouse Down {
        n117 = event-data() -> ("Mods.Double Click"=w251:bool, "CtlRef"=w250:refnum<vi>)  [unwired: 1 in]
        n118 = case shown="True" w251 {
          tunnel: w250 -> [_ w257]
          frame False {
          }
          frame True {
            n119 = property class="Clust"(reference=w257) -> ("Value"=w256:variant)  [unwired: 1 in, 2 out]
            n120 = call "FTW-Reflection-Cluster.vi"("Cluster"=w256) -> ("Cluster Elements"=w255:T33)  [unwired: 14 in]
            n121 = for {
              tunnel: w255 -> [w262] mode=indexing
              tunnel: [w261] -> w254
              stop <- w260 stop-if-true
              n122 = Unbundle By Name(w262) -> ("Element Type"=w259:T32, "Element Value"=w261:variant)
              n123 = Equal?(x=FTW-Reflection-Types."VIReference", y=w259) -> (x = y?=w260:bool)
            }
            n124 = Variant To Data(type=refnum<vi> refnum ("reference"), Variant=w254) -> (data=w252:refnum<vi>)  [unwired: 1 in, 1 out]
            n125 = invoke class="VI" method="FP.Open"(reference=w252) -> ()  [unwired: 4 in, 5 out]
          }
        }
      }
      event Mouse Down {
        n126 = event-data() -> ("Mods.Double Click"=w264:bool, "CtlRef"=w263:refnum<vi>)  [unwired: 1 in]
        n127 = case shown="True" w264 {
          tunnel: w263 -> [_ w270]
          frame False {
          }
          frame True {
            n128 = property class="Clust (strict)"(reference=w270) -> ("Value"=w269:T34)  [unwired: 1 in, 2 out]
            n129 = Unbundle By Name(w269) -> ("CLFNRef"=w268:refnum<vi>)
            n130 = property class="CallLib"(reference=w268) -> ("OwningVI"=w267:refnum<vi>)  [unwired: 1 in, 2 out]
            n131 = property class="VI"(reference=w267, "BDWin.Open"=TRUE ("Block Diagram Window:Open")) -> (error out=w265:errorcluster)  [unwired: 1 in, 1 out]
            n132 = invoke class="CallLib" method="ObjHighlight"(reference=w268, error in=w265) -> ()  [unwired: 1 in, 3 out]
          }
        }
      }
      event "Order By", "Context Filter": Value Change {
        n133 = event-data() -> ()  [unwired: 1 in, 1 out]
        n134 = case shown="\"Execution Settings\"" "Order By" {
          tunnel: w277 -> [w283 w293 w303 w313 w323 w333 w343 w353]
          tunnel: [w282 w292 w302 w312 w322 w332 w342 w352] -> w275
          frame "Application Context" {
            n135 = for {
              tunnel: w283 -> [w291] mode=indexing
              tunnel: [w290] -> w285 mode=indexing
              n136 = Unbundle By Name(w291) -> ("Context"=w289:string, "Name"=w288:string)
              n137 = Bundle("Context"=w289, "Name"=w288, "VIDetails"=w291) -> (w290:T35)  [unwired: 1 in]
            }
            n138 = Sort 1D Array(array=w285) -> (sorted array=w284:T36)
            n139 = for {
              tunnel: w284 -> [w287] mode=indexing
              tunnel: [w286] -> w282 mode=indexing
              n140 = Unbundle(w287) -> ("VIDetails"=w286:T23)  [unwired: 2 out]
            }
          }
          frame "Num Callers" {
            n141 = for {
              tunnel: w293 -> [w301] mode=indexing
              tunnel: [w300] -> w295 mode=indexing
              n142 = Unbundle By Name(w301) -> ("NumCallers"=w299:i32, "Name"=w298:string)
              n143 = Bundle("NumCallers"=w299, "Name"=w298, "VIDetails"=w301) -> (w300:T37)  [unwired: 1 in]
            }
            n144 = Sort 1D Array(array=w295) -> (sorted array=w294:T38)
            n145 = for {
              tunnel: w294 -> [w297] mode=indexing
              tunnel: [w296] -> w292 mode=indexing
              n146 = Unbundle(w297) -> ("VIDetails"=w296:T23)  [unwired: 2 out]
            }
          }
          frame "Complexity" {
            n147 = for {
              tunnel: w303 -> [w311] mode=indexing
              tunnel: [w310] -> w305 mode=indexing
              n148 = Unbundle By Name(w311) -> ("Complexity"=w309:sgl, "CodeSize"=w308:u32)
              n149 = Bundle("Complexity"=w309, "CodeSize"=w308, "VIDetails"=w311) -> (w310:T39)  [unwired: 1 in]
            }
            n150 = Sort 1D Array(array=w305) -> (sorted array=w304:T40)
            n151 = for {
              tunnel: w304 -> [w307] mode=indexing
              tunnel: [w306] -> w302 mode=indexing
              n152 = Unbundle(w307) -> ("VIDetails"=w306:T23)  [unwired: 2 out]
            }
          }
          frame "Diagram Size" {
            n153 = for {
              tunnel: w313 -> [w321] mode=indexing
              tunnel: [w320] -> w315 mode=indexing
              n154 = Unbundle By Name(w321) -> ("CodeSize"=w319:u32, "FPSize"=w318:u32)
              n155 = Bundle("CodeSize"=w319, "FPSize"=w318, "VIDetails"=w321) -> (w320:T41)  [unwired: 1 in]
            }
            n156 = Sort 1D Array(array=w315) -> (sorted array=w314:T42)
            n157 = for {
              tunnel: w314 -> [w317] mode=indexing
              tunnel: [w316] -> w312 mode=indexing
              n158 = Unbundle(w317) -> ("VIDetails"=w316:T23)  [unwired: 2 out]
            }
          }
          frame "FP Size" {
            n159 = for {
              tunnel: w323 -> [w331] mode=indexing
              tunnel: [w330] -> w325 mode=indexing
              n160 = Unbundle By Name(w331) -> ("FPSize"=w329:u32, "CodeSize"=w328:u32)
              n161 = Bundle("FPSize"=w329, "CodeSize"=w328, "VIDetails"=w331) -> (w330:T43)  [unwired: 1 in]
            }
            n162 = Sort 1D Array(array=w325) -> (sorted array=w324:T44)
            n163 = for {
              tunnel: w324 -> [w327] mode=indexing
              tunnel: [w326] -> w322 mode=indexing
              n164 = Unbundle(w327) -> ("VIDetails"=w326:T23)  [unwired: 2 out]
            }
          }
          frame "Compile Time" {
            n165 = for {
              tunnel: w333 -> [w341] mode=indexing
              tunnel: [w340] -> w335 mode=indexing
              n166 = Unbundle By Name(w341) -> ("CompileTime"=w339:i32, "Name"=w338:string)
              n167 = Bundle("CompileTime"=w339, "Name"=w338, "VIDetails"=w341) -> (w340:T45)  [unwired: 1 in]
            }
            n168 = Sort 1D Array(array=w335) -> (sorted array=w334:T46)
            n169 = for {
              tunnel: w334 -> [w337] mode=indexing
              tunnel: [w336] -> w332 mode=indexing
              n170 = Unbundle(w337) -> ("VIDetails"=w336:T23)  [unwired: 2 out]
            }
          }
          frame "Revisions" {
            n171 = for {
              tunnel: w343 -> [w351] mode=indexing
              tunnel: [w350] -> w345 mode=indexing
              n172 = Unbundle By Name(w351) -> ("HistoryRevision"=w349:u32, "Name"=w348:string)
              n173 = Bundle("HistoryRevision"=w349, "Name"=w348, "VIDetails"=w351) -> (w350:T47)  [unwired: 1 in]
            }
            n174 = Sort 1D Array(array=w345) -> (sorted array=w344:T48)
            n175 = for {
              tunnel: w344 -> [w347] mode=indexing
              tunnel: [w346] -> w342 mode=indexing
              n176 = Unbundle(w347) -> ("VIDetails"=w346:T23)  [unwired: 2 out]
            }
          }
          frame "Execution Settings" {
            n177 = for {
              tunnel: w353 -> [w361] mode=indexing
              tunnel: [w360] -> w355 mode=indexing
              n178 = Unbundle By Name(w361) -> ("Execution"=w359:string, "Name"=w358:string)
              n179 = Bundle("Execution"=w359, "Name"=w358, "VIDetails"=w361) -> (w360:T49)  [unwired: 1 in]
            }
            n180 = Sort 1D Array(array=w355) -> (sorted array=w354:T50)
            n181 = for {
              tunnel: w354 -> [w357] mode=indexing
              tunnel: [w356] -> w352 mode=indexing
              n182 = Unbundle(w357) -> ("VIDetails"=w356:T23)  [unwired: 2 out]
            }
          }
        }
        n183 = Concatenate Strings("(?ismx)" ("string"), "Context Filter") -> (w272:string)
        n184 = for {
          tunnel: w275 -> [w281] mode=indexing
          tunnel: [w281] -> w274 mode=indexing if=w280
          tunnel: w272 -> [w279]
          n185 = Unbundle By Name(w281) -> ("Context"=w278:string)
          n186 = call "FTW-Regex.vi"("Regular Expression"=w279, "Input String"=w278) -> ("Match Found?"=w280:bool)  [unwired: 9 in, 4 out]
        }
        "VIs" <- w274
      }
      event "OrderByDocs", "ContextFilterDocs": Value Change {
        n187 = event-data() -> ()  [unwired: 1 in, 1 out]
        n188 = case shown="\"Total Terminals\"" "OrderByDocs" {
          tunnel: w364 -> [w374 w384 w395 w410 w425]
          tunnel: [w373 w383 w394 w409 w424] -> w368
          frame "Name" {
            n189 = for {
              tunnel: w374 -> [w382] mode=indexing
              tunnel: [w381] -> w376 mode=indexing
              n190 = Unbundle By Name(w382) -> ("Context"=w380:string, "Name"=w379:string)
              n191 = Bundle("Context"=w380, "Name"=w379, "VIDocs"=w382) -> (w381:T51)  [unwired: 1 in]
            }
            n192 = Sort 1D Array(array=w376) -> (sorted array=w375:T52)
            n193 = for {
              tunnel: w375 -> [w378] mode=indexing
              tunnel: [w377] -> w373 mode=indexing
              n194 = Unbundle(w378) -> ("VIDocs"=w377:T24)  [unwired: 2 out]
            }
          }
          frame "ConPane Style" {
            n195 = for {
              tunnel: w384 -> [w393] mode=indexing
              tunnel: [w392] -> w386 mode=indexing
              n196 = Unbundle By Name(w393) -> ("ConPane"=w391:u32, "Context"=w390:string, "Name"=w389:string)
              n197 = Bundle("ConPane"=w391, "Context"=w390, "Name"=w389, "VIDocs"=w393) -> (w392:T53)  [unwired: 1 in]
            }
            n198 = Sort 1D Array(array=w386) -> (sorted array=w385:T54)
            n199 = for {
              tunnel: w385 -> [w388] mode=indexing
              tunnel: [w387] -> w383 mode=indexing
              n200 = Unbundle(w388) -> ("VIDocs"=w387:T24)  [unwired: 3 out]
            }
          }
          frame "Required Terminals" {
            n201 = for {
              tunnel: w395 -> [w408] mode=indexing
              tunnel: [w407] -> w397 mode=indexing
              n202 = Unbundle By Name(w408) -> ("InReq"=w405:u32, "OutReq"=w403:u32, "InRec"=w402:u32, "OutRec"=w401:u32, "Name"=w406:string)
              n203 = Add(x=w402, y=w401) -> (x+y=w400:u32)
              n204 = Add(x=w405, y=w403) -> (x+y=w404:u32)
              n205 = Bundle(w404, w400, "Name"=w406, "VIDocs"=w408) -> (w407:T55)  [unwired: 1 in]
            }
            n206 = Sort 1D Array(array=w397) -> (sorted array=w396:T56)
            n207 = for {
              tunnel: w396 -> [w399] mode=indexing
              tunnel: [w398] -> w394 mode=indexing
              n208 = Unbundle(w399) -> ("VIDocs"=w398:T24)  [unwired: 3 out]
            }
          }
          frame "Recommended Terminals" {
            n209 = for {
              tunnel: w410 -> [w423] mode=indexing
              tunnel: [w422] -> w412 mode=indexing
              n210 = Unbundle By Name(w423) -> ("InRec"=w420:u32, "OutRec"=w418:u32, "InReq"=w417:u32, "OutReq"=w416:u32, "Name"=w421:string)
              n211 = Add(x=w417, y=w416) -> (x+y=w415:u32)
              n212 = Add(x=w420, y=w418) -> (x+y=w419:u32)
              n213 = Bundle(w419, w415, "Name"=w421, "VIDocs"=w423) -> (w422:T55)  [unwired: 1 in]
            }
            n214 = Sort 1D Array(array=w412) -> (sorted array=w411:T56)
            n215 = for {
              tunnel: w411 -> [w414] mode=indexing
              tunnel: [w413] -> w409 mode=indexing
              n216 = Unbundle(w414) -> ("VIDocs"=w413:T24)  [unwired: 3 out]
            }
          }
          frame "Total Terminals" {
            n217 = for {
              tunnel: w425 -> [w431] mode=indexing
              tunnel: [w433] -> w427 mode=indexing
              n218 = Unbundle By Name(w431) -> ("Wired Terms"=w430:u32, "Name"=w432:string)
              n219 = Bundle("Wired Terms"=w430, "Name"=w432, "VIDocs"=w431) -> (w433:T57)  [unwired: 1 in]
            }
            n220 = Sort 1D Array(array=w427) -> (sorted array=w426:T58)
            n221 = for {
              tunnel: w426 -> [w429] mode=indexing
              tunnel: [w428] -> w424 mode=indexing
              n222 = Unbundle(w429) -> ("VIDocs"=w428:T24)  [unwired: 2 out]
            }
          }
        }
        n223 = Concatenate Strings("(?ismx)" ("string"), "ContextFilterDocs") -> (w366:string)
        n224 = for {
          tunnel: w368 -> [w372] mode=indexing
          tunnel: [w372] -> w362 mode=indexing if=w371
          tunnel: w366 -> [w370]
          n225 = Unbundle By Name(w372) -> ("Context"=w369:string)
          n226 = call "FTW-Regex.vi"("Regular Expression"=w370, "Input String"=w369) -> ("Match Found?"=w371:bool)  [unwired: 9 in, 4 out]
        }
        "VIDocs" <- w362
      }
      event "Check Coverage": Value Change {
        n227 = event-data() -> ()  [unwired: 1 in, 1 out]
        n228 = invoke class="App" method="CodeCov.AllVIs"("contextName"=w436) -> ("measuredVIs"=w437:path[])  [unwired: 4 in, 4 out]
        n229 = for {
          tunnel: w437 -> [w442] mode=indexing
          tunnel: w436 -> [w443]
          tunnel: [w438] -> w435 mode=indexing
          n230 = invoke class="App" method="CodeCov.VIPercentage"("contextName"=w443, "covPercent"=w442) -> ("covPercent"=w440:dbl, "infoFound"=w441:bool)  [unwired: 5 in, 5 out]
          n231 = Format Into String(w442) -> (resulting string=w439:string)  [unwired: 3 in, 1 out]
          n232 = Bundle("infoFound"=w441, "covPercent"=w440, w439) -> (w438:T59)  [unwired: 1 in]
        }
        n233 = Sort 1D Array(array=w435) -> (sorted array=→"Array":T60)
      }
      event "ExtendedLinkerInfo": Mouse Move {
        w455 = 3 ("x")
        n234 = event-data() -> ("Coords.Horizontal"=w461:i32)  [unwired: 1 in]
        n235 = property on="Flags" class="Arr (strict)"() -> ("Left"=w453:i32, "Width"=w454:u32, "Number of Columns"=w459:u32)  [unwired: 2 in, 2 out]
        n236 = To Long Integer(number=w454) -> (32bit integer=w448:i32)
        n237 = To Long Integer(number=w459) -> (32bit integer=w447:i32)
        n238 = Multiply(x=w455, y=2) -> (x*y=w457:i32)
        n239 = Add(x=w455, y=w453) -> (x+y=w451:i32)
        n240 = Subtract(x=w448, y=w457) -> (x-y=w458:i32)
        n241 = Quotient & Remainder(x=w458, y=w447) -> (floor(x/y)=w452:i32)  [unwired: 1 out]
        n242 = Subtract(x=w461, y=w451) -> (x-y=w460:i32)
        n243 = Quotient & Remainder(x=w460, y=w452) -> (floor(x/y)=w449:i32)  [unwired: 1 out]
        n244 = Index Array(array=w450, index=w449) -> (element=w446:string)
        n245 = Format Into String(format string="%s", w446) -> (resulting string=→"Hover Tip":string)  [unwired: 2 in, 1 out]
      }
    }
  }
  n246 = for {
    N -> [w465]
    tunnel: w17 -> [w473] mode=indexing
    tunnel: [w476] -> w16 mode=indexing
    tunnel: [w468] -> w14 mode=concatenating
    tunnel: [w463] -> w11 mode=concatenating
    i -> [w466]
    n247 = Increment(x=w466) -> (x+1=w467:i32)
    n248 = Unbundle By Name(w473) -> ("Filetype"=w475:T10, "delimited name"=w469:string)
    n249 = Divide(x=w467, y=w465) -> (x/y=→"CLFN Progress...":dbl)
    n250 = call "FTW-Linker-DecodeBitmap.vi"("LinkerInfo"=w473) -> ("All Flags"=w472:bool[])  [unwired: 8 in, 6 out]
    n251 = Format Into String(w475) -> (resulting string=w474:string)  [unwired: 3 in, 1 out]
    n252 = Open VI Reference(vi path=w469) -> (vi reference=w471:refnum<vi>)  [unwired: 5 in, 1 out]
    n253 = case shown="True" "ScanCLFN" {
      tunnel: w471 -> [w477 w487]
      tunnel: [w477 w486] -> w470
      tunnel: w469 -> [_ w483]
      tunnel: [_ w482] -> w468
      tunnel: [_ w480] -> w463
      frame False {
      }
      frame True {
        w478 = refnum<vi> refnum ("GObject")
        n254 = property class="VI"(reference=w487) -> (reference out=w486:refnum<vi>, "Diagram"=w481:refnum<vi>)  [unwired: 1 in, 1 out]
        n255 = disable-structure shown="Disabled" {
          disable-tunnel: [w488 _] -> w479
          frame Disabled {
            n256 = local read "CLFNs"() -> (w489:T8)
            n257 = Index Array(array=w489) -> (element=w488:T34)  [unwired: 1 in]
          }
          frame Enabled {
          }
        }
        n258 = call "FTW-CodeGen-FindGObjects.vi"("GObject to Traverse"=w481, "Class Type Reference"=w478) -> ("GObject Instances"=w485:refnum<vi>[], "error out"=w484:errorcluster)  [unwired: 12 in]
        n259 = for {
          tunnel: w485 -> [w518] mode=indexing
          tunnel: w478 -> [w517]
          tunnel: w484 -> [w516]
          tunnel: w483 -> [w514]
          tunnel: [w513] -> w482 mode=indexing
          tunnel: w479 -> [w512]
          tunnel: [w490] -> w480 mode=indexing
          n260 = To More Specific Class(target class=w517, reference=w518, error in=w516) -> (specific class reference=w500:refnum<vi>, error out=w515:errorcluster)
          n261 = property class="CallLib"(reference=w500, error in=w515) -> (reference out=w503:refnum<vi>, error out=w496:errorcluster, "FuncName"=w492:string, "CallConvention"=w511:u32, "LibPath"=w510:path, "Re-entrant"=w508:bool, "DynamicLib"=w509:bool, "ErrorCheckingLevel"=w507:u32, "ReserveCallback"=w506:string, "UnreserveCallback"=w505:string, "AbortCallback"=w504:string, "Allow Prealloc"=w499:bool[])
          n262 = invoke class="CallLib" method="Prototype"(reference=w503, "typedefs?"=FALSE ("Include Typedefs?")) -> (reference out=w502:refnum<vi>, error out=w494:errorcluster, "Proto"=w498:string)  [unwired: 4 in, 3 out]
          n263 = Merge Errors(w496, w494) -> (w495:errorcluster)
          n264 = call "FTW-ERR-SerializeForLog.vi"("error in"=w495) -> ("Serialized Error"=w493:string)
          n265 = call "FTW-STR-ReplaceWhitespace.vi"("Replace Spaces With..."=" ", "Input"=w498) -> ("Output"=w491:string)  [unwired: 2 in]
          n266 = Bundle(cluster=w512, "CLFNRef"=w502, "VI"=w514, "Function"=w492, "Prototype"=w491, "CallConv"=w511, "LibraryPath"=w510, "AnyThread"=w508, "Dynamic"=w509, "ErrCheckLevel"=w507, "Reserve"=w506, "Unreserve"=w505, "Abort"=w504, "Prealloc"=w499, "Err"=w493) -> (w513:T34)
          n267 = Bundle("FuncName"=w492, "Output"=w491) -> (w490:cluster{"FuncName":string, "Output":string})  [unwired: 1 in]
        }
      }
    }
    n268 = Bundle(w474, "delimited name"=w469, "All Flags"=w472, "vi reference"=w470) -> (w476:T61)  [unwired: 1 in]
  }
  n269 = for {
    tunnel: w14 -> [w523] mode=indexing
    tunnel: [w522] -> w71 mode=indexing
    n270 = Unbundle By Name(w523) -> ("LibraryPath"=w519:path, "VI"=w520:string, "Function"=w521:string)
    n271 = Bundle("LibraryPath"=w519, "VI"=w520, "Function"=w521, "CLFN Array Element"=w523) -> (w522:T62)  [unwired: 1 in]
  }
  n272 = Sort 1D Array(array=w11) -> (sorted array=w10:cluster{"FuncName":string, "Output":string}[])
  n273 = Sort 1D Array(array=w16) -> (sorted array=→"ExtendedLinkerInfo":T63)
  n274 = for {
    tunnel: w10 -> [w525] mode=indexing
    tunnel: [w524] -> w9 mode=indexing
    n275 = Unbundle(w525) -> ("Output"=w524:string)  [unwired: 1 out]
  }
  n276 = call "FTW-STR-Array-Delimit.vi"("Array of Strings"=w9, "Delimiter"="\n\n") -> ("Delimited String"=→"All Prototypes":string)  [unwired: 13 in]
  n277 = Sort 1D Array(array=w71) -> (sorted array=w72:T64)
  n278 = for {
    tunnel: w72 -> [w527] mode=indexing
    tunnel: [w526] -> w70 mode=indexing
    n279 = Unbundle(w527) -> ("CLFN Array Element"=w526:T34)  [unwired: 3 out]
  }
  "CLFNs" <- w70
